vi "Write String.vi"(8 "error in (no error)":errorcluster, 10 "String":string, 11 "Alpaca Tokenizer in":refnum<class "Lexer.lvclass">) -> (0 "error out":errorcluster, 3 "Alpaca Tokenizer out":refnum<class "Lexer.lvclass">)   [LabVIEW 2019, in "JKI JSON Serialization.lvlib" / "Lexer.lvclass"]
doc: "JKI JSON 1.1.10.37\nTomi Maila - JKI\nCopyright (c) 2017, JKI"
uses:
  Lexer.lvclass
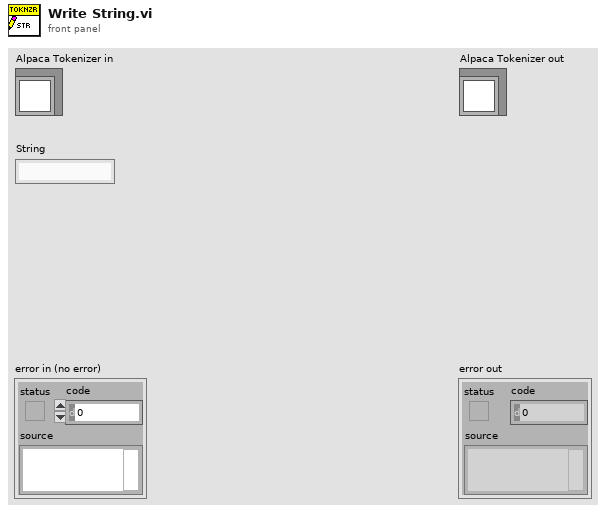
[diagram p1: front panel]
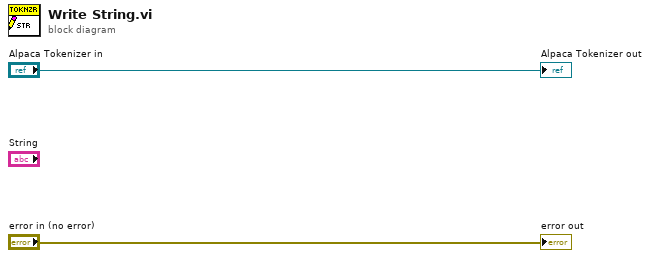
[diagram p0: block diagram]
diagram:
  "error out" <- "error in (no error)"
  "Alpaca Tokenizer out" <- "Alpaca Tokenizer in"
